vi "Table Set Header Name and Data (DBL).vi"(7 "format string":string="%.3p", 9 "Data":dbl[][](array[numeric]), 10 "Header":string[](array[string]), 11 "Table Ref":refnum<vi>) -> ()   [LabVIEW 2023, in "FPT Pulse Measurement UI.lvlib"]
uses:
  FPT Pulse Measurement UI.lvlib
panel:
  out "Array":string[][](array[string])
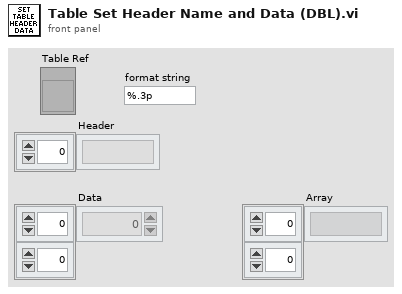
[diagram p1: front panel]
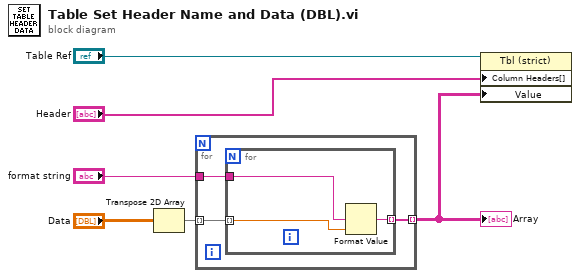
[diagram p0: block diagram]
diagram:
  n1 = Transpose 2D Array(2D array="Data") -> (transposed array=w6:dbl[][])
  n2 = for {
    tunnel: w6 -> [w9] mode=indexing
    tunnel: [w8] -> w2 mode=indexing
    tunnel: "format string" -> [w7]
    n3 = for {
      tunnel: w9 -> [w12] mode=indexing
      tunnel: [w11] -> w8 mode=indexing
      tunnel: w7 -> [w10]
      n4 = Format Value(format string=w10, value (0)=w12) -> (output string=w11:string)  [unwired: 1 in]
    }
  }
  "Array" <- w2
  n5 = property on="Property Node" class="Tbl (strict)"(reference="Table Ref", "Column Headers[]"="Header", "Value"=w2) -> ()  [unwired: 1 in, 2 out]
